vi "Tester_oop.vi"(8 "error in (no error)":errorcluster) -> (0 "error out":errorcluster)   [LabVIEW 2020]
uses:
  Typedefs/XY Stage config cluster.ctl
  Typedefs/XYZ channel ring.ctl
  typedefs/TranslationStageControlInfo.ctl
  Generic Comms/CommsProtocol/CommsProtocol.lvclass
  typedefs/XYZControlConfig.ctl
  Serial Comms/Serial Comms/Serial Comms.lvclass
  C:/LV_unversioned_SP/local_copy_ml_yale/Peripherals Control/Generic Comms/CommsProtocol/CommsProtocol.lvclass
  Serial Comms/Serial - Settings.ctl
  XYZ Stage Control/XYZ Stage Control.lvclass
  Scientifica XYZ Gen1/Scientifica XYZ Gen1.lvclass
  XYZ Stage Control/typedefs/XYZ_position_input.ctl
  XYZ Stage Control/typedefs/XYZ axes.ctl
  Typedefs/XYZ_coordinates.ctl
panel:
  in  "Z":bool
  in  "Y":bool
  in  "X":bool
  in  "move step":dbl
  in  "Channel":T1="Z"
  in  "Reset axes":bool
  in  "class factory":bool
  out "error live":errorcluster
  out "No Feedback":bool
  out "x-y":u32
  out "comms init ?":bool
  out "Stage XYZ Position":cluster{"X":sgl, "Y":sgl, "Z":sgl}
  in  "Read Position":bool
  in  "XY Stage":T2
  out "file or folder exists?":bool
  out "appended path":path
  out "Application Directory":path
  in  "Stagetype":enum16{"Scientifica", "Other"}(ring)
  in  "Exit":bool
  in  "Initialize":bool
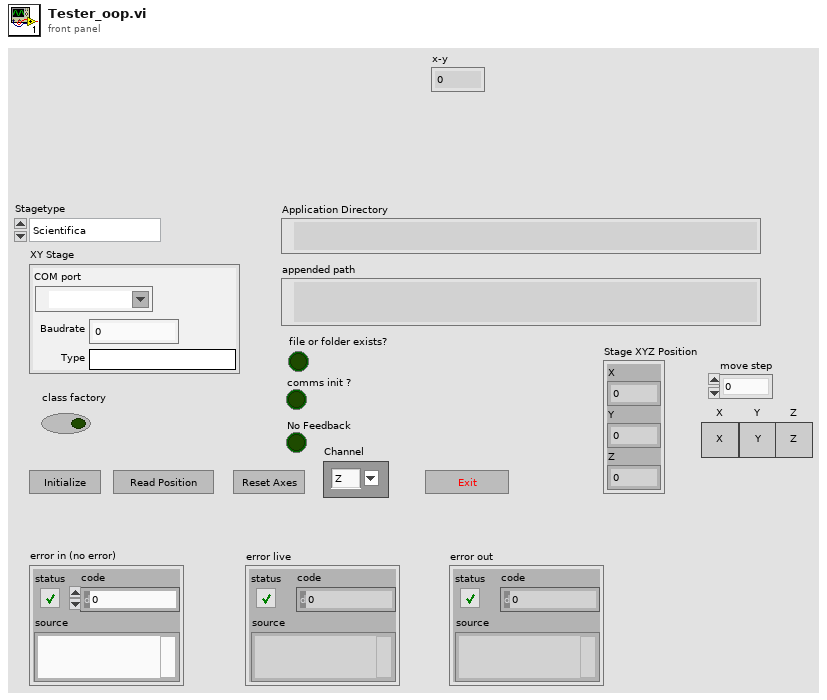
[diagram p1: front panel]
types:
  T1 = typedef "XYZ channel ring.ctl" = string
  T2 = typedef "XY Stage config cluster.ctl" = cluster{"COM port":refnum<visa-resource-name>, "Baudrate":i32, "Type":string}
  T3 = typedef "Serial - Settings.ctl" = cluster{"VISA resource name ":refnum<visa-resource-name>, "baud rate":u32, "data bits":u16, "parity":enum16{"None", "Odd", "Even", "Mark", "Space"}, "stop bits":u16, "flow control":u16, "Timeout":u32, "termination char\n(0xA = '\\n' = LF) ":u8, "Enable Termination Character":bool}
  T4 = typedef "XYZControlConfig.ctl" = enum16{"None", "XYZ", "XY-Z", "X-Y-Z", "Z"}
  T5 = typedef "TranslationStageControlInfo.ctl" = cluster{"CommsProtocol.lvclass":refnum<class "CommsProtocol.lvclass">, "CommsProtocol.lvclass 2":refnum<class "CommsProtocol.lvclass">, "CommsProtocol.lvclass 3":refnum<class "CommsProtocol.lvclass">, "XYZ Control Config":T4, "Translation Stage Description":string}
  T6 = typedef "XYZ_position_input.ctl" = cluster{"Speed":i32, "Z Limit (um+/-)":sgl, "Axes":T7, "XYZ Coordinates":T8}
  T7 = typedef "XYZ axes.ctl" = string
  T8 = typedef "XYZ_coordinates.ctl" = cluster{"X":sgl, "Y":sgl, "Z":sgl}
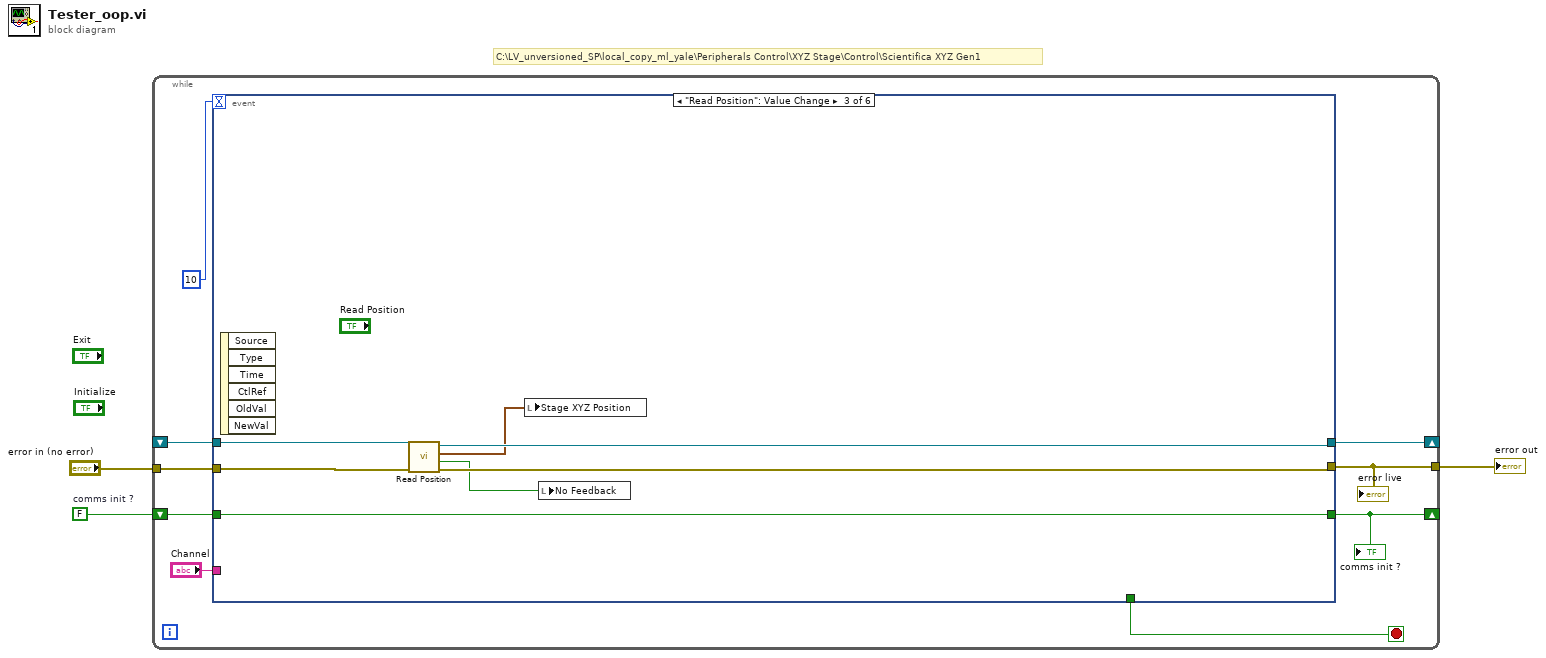
[diagram p0: block diagram]
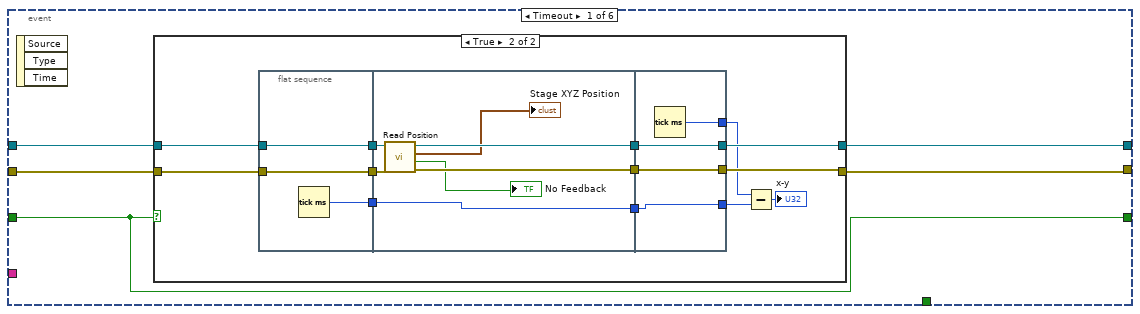
[diagram p2: hidden frame]
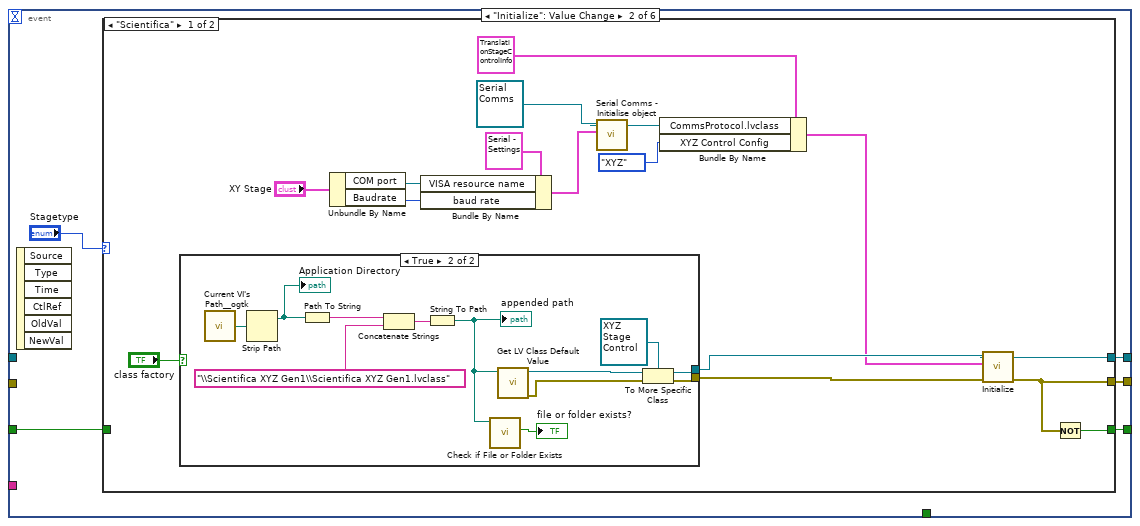
[diagram p4: hidden frame]
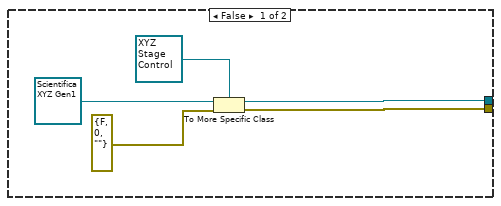
[diagram p5: hidden frame]
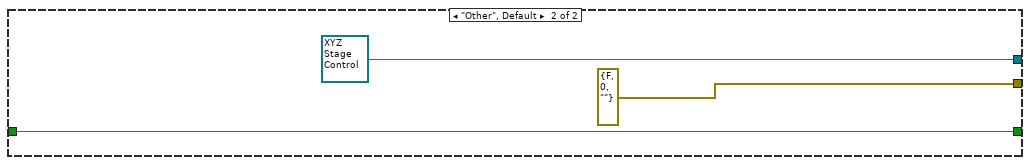
[diagram p6: hidden frame]
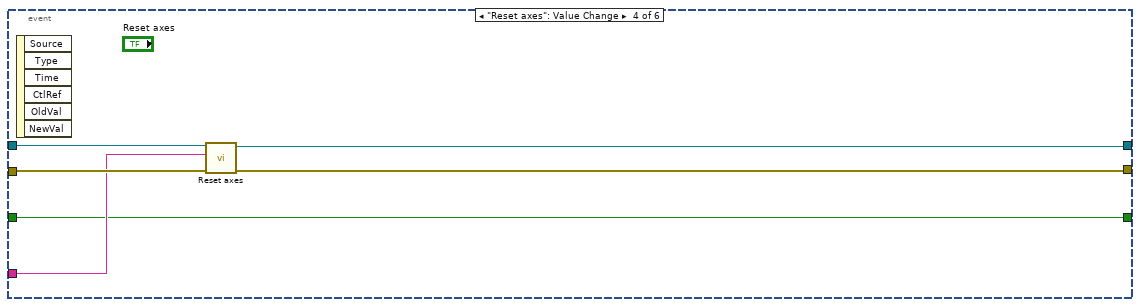
[diagram p7: hidden frame]
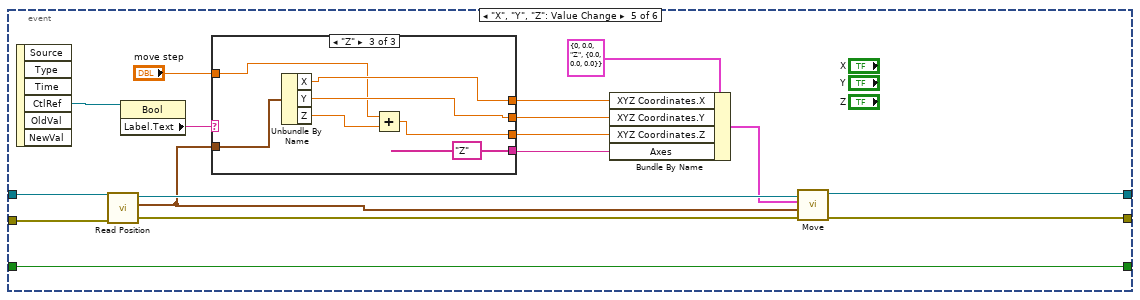
[diagram p8: hidden frame]
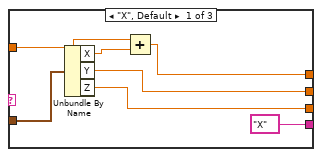
[diagram p9: hidden frame]
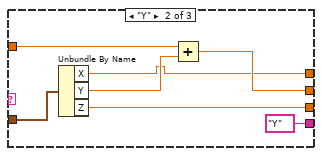
[diagram p10: hidden frame]
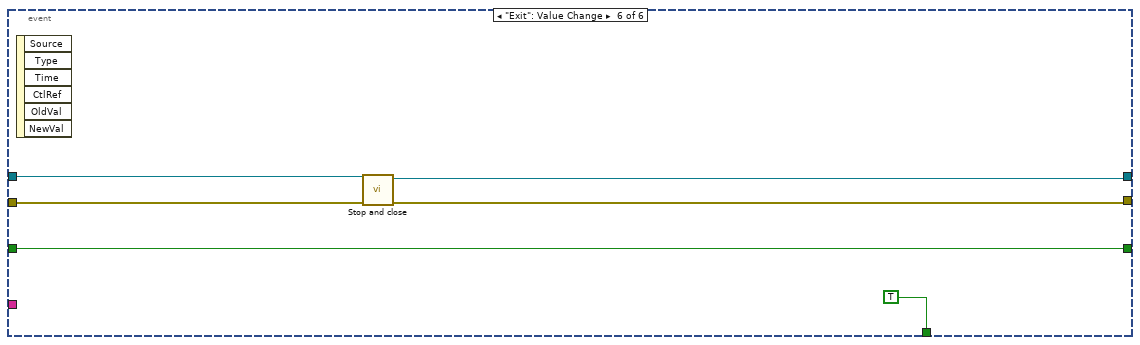
[diagram p11: hidden frame]
diagram:
  w1 = FALSE  # comms init ?
  # "C:\\LV_unversioned_SP\\local_copy_ml_yale\\Peripherals Control\\XYZ Stage\\Control\\Scientifica XYZ Gen1"
  n1 = while {
    tunnel: [w11] -> w3
    shift-right: [w10] -> _
    shift-left: _ -> [w9]
    tunnel: "error in (no error)" -> [w8]
    shift-right: [w5] -> _
    shift-left: w1 -> [w6]
    stop <- w7 stop-if-true
    n2 = event shown="[2] \"Read Position\": Value Change" {
      selector: _ -> [_ _ _ _ _ _]
      dyn-events: _ -> [_ _ _ _ _ _]
      timeout: 10 -> [_ _ _ _ _ _]
      tunnel: [w14 w50 w91 w99 w103 w139] -> w11
      tunnel: [w15 w49 w92 w97 w104 w140] -> w10
      tunnel: w9 -> [w17 _ w94 w98 w114 w141]
      tunnel: w8 -> [w16 _ w93 w100 w115 w142]
      tunnel: [_ _ _ _ _ TRUE] -> w7
      tunnel: w6 -> [w13 w48 w90 w95 w102 w143]
      tunnel: [w13 w47 w90 w95 w102 w143] -> w5
      tunnel: "Channel" -> [_ _ _ w96 _ _]
      event Timeout {
        n3 = event-data() -> ()  [unwired: 1 in, 3 out]
        n4 = case shown="True" w13 {
          tunnel: w17 -> [w19 w32]
          tunnel: w16 -> [w18 w31]
          tunnel: [w19 w30] -> w15
          tunnel: [w18 w29] -> w14
          frame False {
          }
          frame True {
            n5 = flat-sequence {
              tunnel: w31 -> [w34]
              tunnel: w32 -> [w35]
              tunnel: [w35] -> w28
              tunnel: [w34] -> w27
              tunnel: [w33] -> w22
              tunnel: w28 -> [w42]
              tunnel: w27 -> [w41]
              tunnel: [w40] -> w26
              tunnel: [w39] -> w25
              tunnel: [w37] -> w23
              tunnel: w22 -> [w37]
              tunnel: [w45] -> w29
              tunnel: [w46] -> w30
              tunnel: w26 -> [w46]
              tunnel: w25 -> [w45]
              tunnel: [w44] -> w24
              tunnel: w23 -> [w43]
              tunnel: [w43] -> w21
              frame #0 {
                n6 = Tick Count (ms)() -> (millisecond timer value=w33:u32)
              }
              frame #1 {
                n7 = call-dynamic "Read Position.vi"("error in (no error)"=w41, "XYZ Stage Control in"=w42) -> ("error out"=w39:errorcluster, "No Feedback"=→"No Feedback":bool, "Stage XYZ Position"=→"Stage XYZ Position":cluster{"X":sgl, "Y":sgl, "Z":sgl}, "XYZ Stage Control out"=w40:refnum<class "XYZ Stage Control.lvclass">)  [unwired: 6 in]
              }
              frame #2 {
                n8 = Tick Count (ms)() -> (millisecond timer value=w44:u32)
              }
            }
            n9 = Subtract(x=w24, y=w21) -> (x-y=→"x-y":u32)
          }
        }
      }
      event "Initialize": Value Change {
        n10 = event-data() -> ()  [unwired: 1 in, 6 out]
        n11 = case shown="\"Scientifica\"" "Stagetype" {
          tunnel: [w64 errorcluster {"status"=FALSE, "code"=0, "source"=""} ("error out")] -> w50
          tunnel: [w65 refnum<class "XYZ Stage Control.lvclass"> refnum ("XYZ Stage Control.lvclass")] -> w49
          tunnel: w48 -> [_ w85]
          tunnel: [w63 w85] -> w47
          frame "Scientifica" {
            n12 = case shown="True" "class factory" {
              tunnel: [w68 w81] -> w67
              tunnel: [w69 w80] -> w66
              frame False {
                n13 = To More Specific Class(target class=refnum<class "XYZ Stage Control.lvclass"> refnum ("XYZ Stage Control.lvclass"), reference=refnum<class "Scientifica XYZ Gen1.lvclass"> refnum ("Scientifica XYZ Gen1.lvclass"), error in=errorcluster {"status"=FALSE, "code"=0, "source"=""}) -> (specific class reference=w69:refnum<class "XYZ Stage Control.lvclass">, error out=w68:errorcluster)
              }
              frame True {
                n14 = call <userlib>:"Current VI's Path__ogtk.vi"() -> ("Current VI's Path (+ Relative)"=w78:path)  [unwired: 1 in]
                n15 = Strip Path(path=w78) -> (stripped path=w77:path)  [unwired: 1 out]
                "Application Directory" <- w77
                n16 = Path To String(path=w77) -> (string=w76:string)
                n17 = Concatenate Strings(w76, "\\Scientifica XYZ Gen1\\Scientifica XYZ Gen1.lvclass") -> (w74:string)
                n18 = String To Path(string=w74) -> (path=w73:path)
                "appended path" <- w73
                n19 = call <vilib>:"Check if File or Folder Exists.vi"("path"=w73) -> ("file or folder exists?"=→"file or folder exists?":bool)  [unwired: 8 in, 2 out]
                n20 = call <vilib>:"Get LV Class Default Value.vi"("class path"=w73) -> ("error out"=w83:errorcluster, "object"=w84:refnum<class>)  [unwired: 9 in]
                n21 = To More Specific Class(target class=refnum<class "XYZ Stage Control.lvclass"> refnum ("XYZ Stage Control.lvclass"), reference=w84, error in=w83) -> (specific class reference=w80:refnum<class "XYZ Stage Control.lvclass">, error out=w81:errorcluster)
              }
            }
            n22 = Unbundle By Name("XY Stage") -> ("COM port"=w53:refnum<visa-resource-name>, "Baudrate"=w52:i32)
            n23 = Bundle By Name(cluster=T3 {"VISA resource name "="", "baud rate"=9600, "data bits"=8, "parity"=enum."None", "stop bits"=10, "flow control"=0, "Timeout"=0, "termination char\n(0xA = '\\n' = LF) "=10, "Enable Termination Character"=FALSE} ("Serial Settings"), "VISA resource name"=w53, "baud rate"=w52) -> (w56:T3)
            n24 = call "Serial Comms - Initialise object.vi"("Serial Settings"=w56, "Serial Comms in"=refnum<class "Serial Comms.lvclass"> refnum ("Serial Comms.lvclass")) -> ("Serial Comms out"=w55:refnum<class "Serial Comms.lvclass">)  [unwired: 8 in, 1 out]
            n25 = Bundle By Name(cluster=T5 {"CommsProtocol.lvclass"=refnum, "CommsProtocol.lvclass 2"=refnum, "CommsProtocol.lvclass 3"=refnum, "XYZ Control Config"=enum."None", "Translation Stage Description"=""} ("Stage Comms"), "CommsProtocol.lvclass"=w55, "XYZ Control Config"=XYZControlConfig."XYZ") -> (w59:T5)
            n26 = call-dynamic "Initialize.vi"("error in (no error)"=w67, "Stage Comms"=w59, "XYZ Stage Control in"=w66) -> ("error out"=w64:errorcluster, "XYZ Stage Control out"=w65:refnum<class "XYZ Stage Control.lvclass">)  [unwired: 7 in]
            n27 = Not(x=w64) -> (.not. x?=w63:bool)
          }
          frame "Other", Default {
          }
        }
      }
      event "Read Position": Value Change {
        n28 = event-data() -> ()  [unwired: 1 in, 6 out]
        n29 = call-dynamic "Read Position.vi"("error in (no error)"=w93, "XYZ Stage Control in"=w94) -> ("error out"=w91:errorcluster, "No Feedback"=w88:bool, "Stage XYZ Position"=w89:cluster{"X":sgl, "Y":sgl, "Z":sgl}, "XYZ Stage Control out"=w92:refnum<class "XYZ Stage Control.lvclass">)  [unwired: 6 in]
        n30 = local write "Stage XYZ Position"(w89) -> ()
        n31 = local write "No Feedback"(w88) -> ()
      }
      event "Reset axes": Value Change {
        n32 = event-data() -> ()  [unwired: 1 in, 6 out]
        n33 = call-dynamic "Reset axes.vi"("error in (no error)"=w100, "Channel"=w96, "XYZ Stage Control in"=w98) -> ("error out"=w99:errorcluster, "XYZ Stage Control out"=w97:refnum<class "XYZ Stage Control.lvclass">)  [unwired: 7 in]
      }
      event "X", "Y", "Z": Value Change {
        n34 = event-data() -> ("CtlRef"=w117:refnum<vi>)  [unwired: 1 in, 5 out]
        n35 = call-dynamic "Read Position.vi"("error in (no error)"=w115, "XYZ Stage Control in"=w114) -> ("error out"=w111:errorcluster, "Stage XYZ Position"=w112:cluster{"X":sgl, "Y":sgl, "Z":sgl}, "XYZ Stage Control out"=w113:refnum<class "XYZ Stage Control.lvclass">)  [unwired: 6 in, 1 out]
        n36 = property class="Bool"(reference=w117) -> ("Label.Text"=w116:string)  [unwired: 1 in, 2 out]
        n37 = case shown="\"Z\"" w116 {
          tunnel: [T1 "X" ("Channel 2") T1 "Y" ("Channel 2") T1 "Z" ("Channel 2")] -> w109
          tunnel: w112 -> [w123 w130 w137]
          tunnel: "move step" -> [w121 w125 w133]
          tunnel: [w120 w127 w136] -> w101
          tunnel: [w119 w128 w135] -> w107
          tunnel: [w118 w126 w132] -> w106
          frame "X", Default {
            n38 = Unbundle By Name(w123) -> ("X"=w122:sgl, "Y"=w119:sgl, "Z"=w118:sgl)
            n39 = Add(x=w121, y=w122) -> (x+y=w120:dbl)
          }
          frame "Y" {
            n40 = Unbundle By Name(w130) -> ("X"=w127:sgl, "Y"=w129:sgl, "Z"=w126:sgl)
            n41 = Add(x=w125, y=w129) -> (x+y=w128:dbl)
          }
          frame "Z" {
            n42 = Unbundle By Name(w137) -> ("X"=w136:sgl, "Y"=w135:sgl, "Z"=w134:sgl)
            n43 = Add(x=w133, y=w134) -> (x+y=w132:dbl)
          }
        }
        n44 = Bundle By Name(cluster=T6 {"Speed"=0, "Z Limit (um+/-)"=0.0, "Axes"="Z", "XYZ Coordinates"={"X"=0.0, "Y"=0.0, "Z"=0.0}} ("XYZ Position Input"), "XYZ Coordinates.X"=w101, "XYZ Coordinates.Y"=w107, "XYZ Coordinates.Z"=w106, "Axes"=w109) -> (w105:T6)
        n45 = call-dynamic "Move.vi"("error in (no error)"=w111, "Current XYZ Position"=w112, "XYZ Position Input"=w105, "XYZ Stage Control in"=w113) -> ("error out"=w103:errorcluster, "XYZ Stage Control out"=w104:refnum<class "XYZ Stage Control.lvclass">)  [unwired: 5 in, 1 out]
      }
      event "Exit": Value Change {
        n46 = event-data() -> ()  [unwired: 1 in, 6 out]
        n47 = call-dynamic "Stop and close.vi"("error in (no error)"=w142, "XYZ Stage Control in"=w141) -> ("error out"=w139:errorcluster, "XYZ Stage Control out"=w140:refnum<class "XYZ Stage Control.lvclass">)  [unwired: 8 in]
      }
    }
    "comms init ?" <- w5
    "error live" <- w11
  }
  "error out" <- w3
